vi "Read Voltage From Channel.vi"(8 "error in (no error)":errorcluster, 10 "Channel":u8, 11 "PXIe-5172:Fetch Waveforms CFG in":refnum<class "Voltmeter CFG.lvclass">=refnum) -> (0 "error out":errorcluster, 2 "Voltage":dbl format="%#_g V", 3 "PXIe-5172:Fetch Waveforms CFG out":refnum<class "Voltmeter CFG.lvclass">)   [LabVIEW 2023, in "PXIe-5172.lvlib" / "Fetch Waveforms CFG.lvclass"]
uses:
  Fetch Waveforms CFG.lvclass
  <vilib>/Analysis/NI_AALBase.lvlib
  <vilib>/Analysis/baseanly.llb/Mean (DBL).vi
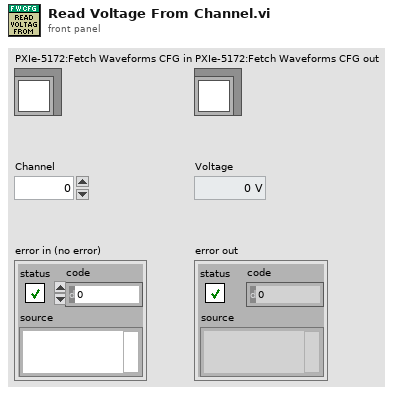
[diagram p1: front panel]
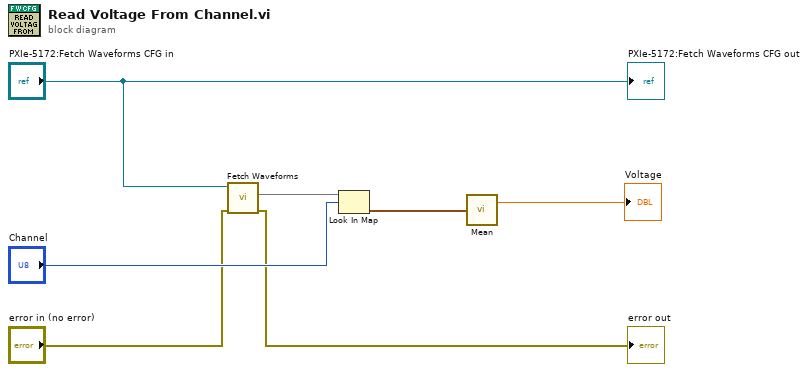
[diagram p0: block diagram]
diagram:
  n1 = call-dynamic "Fetch Waveforms.vi"("error in"="error in (no error)", "object in"="PXIe-5172:Fetch Waveforms CFG in") -> ("error out"=→"error out":errorcluster, "Last Waveforms"=w5:map{u8, waveform(dbl)})  [unwired: 7 in, 1 out]
  n2 = Look In Map(map=w5, key="Channel") -> (value=w3:waveform(dbl))  [unwired: 1 in, 1 out]
  n3 = call-poly <vilib>:"Mean.vi"("X"=w3) -> ("mean"=→"Voltage":dbl)  [unwired: 1 out]
  "PXIe-5172:Fetch Waveforms CFG out" <- "PXIe-5172:Fetch Waveforms CFG in"
